vi "Stereo - IMAQ PrivGetCalibrationImageSampleInfo.vi"(8 "error in (no error)":errorcluster, 9 "Options":T3, 10 "Index":i32, 11 "Template Image":T4) -> (0 "error out":errorcluster, 1 "Undistorted Points":cluster{"X":dbl, "Y":dbl}[](array[cluster]), 2 "Back Projected Points":cluster{"X":dbl, "Y":dbl}[](array[cluster]), 3 "Reference Points":T1, 5 "Euler Angles":cluster{"X":dbl, "Y":dbl, "Z":dbl})   [LabVIEW 2014]
doc: "Returns information on the template image."
uses:
  <vilib>/vision/Image Controls.llb/IMAQ Image.ctl
  <vilib>/vision/Calibration.llb/Calibration Reference Points.ctl
  nivision.dll
panel:
  # "Overview: Returns information on the template image."
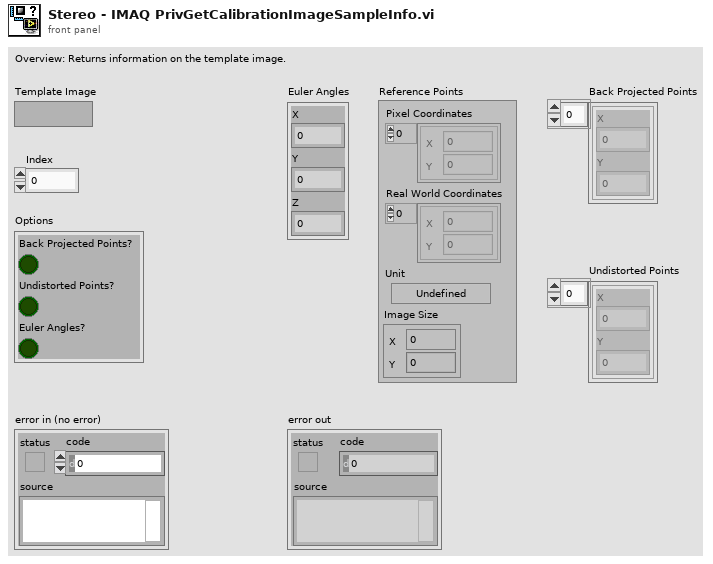
[diagram p1: front panel]
types:
  T1 = typedef "Calibration Reference Points.ctl" = cluster{"Pixel Coordinates":cluster{"X":dbl, "Y":dbl}[], "Real World Coordinates":cluster{"X":dbl, "Y":dbl}[], "Unit":T2, "Image Size":cluster{"X":u32, "Y":u32}}
  T2 = typedef "Image Unit" = enum32{"Undefined", "Angström", "Micrometer", "Millimeter", "Centimeter", "Meter", "Kilometer", "Microinch", "Inch", "Feet", "Nautical miles", "Standard miles", "Steps"}
  T3 = cluster{"Back Projected Points?":bool, "Undistorted Points?":bool, "Euler Angles?":bool}
  T4 = typedef "IMAQ Image.ctl" = refnum<image>
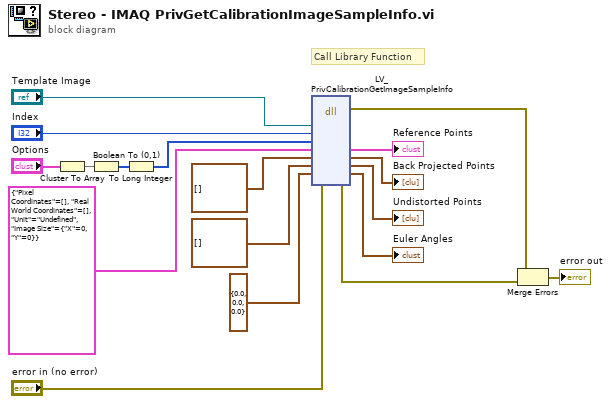
[diagram p0: block diagram]
diagram:
  # "Call Library Function"
  n1 = Cluster To Array(cluster="Options") -> (array=w9:bool[])
  n2 = Boolean To (0,1)(Boolean=w9) -> (0, 1=w7:i16[])
  n3 = To Long Integer(number=w7) -> (32bit integer=w6:i32[])
  n4 = dll-call lib="nivision.*" fn="LV_PrivCalibrationGetImageSampleInfo"("srcImage"="Template Image", "index"="Index", "options"=w6, "pixel points"=T1 {"Pixel Coordinates"=[], "Real World Coordinates"=[], "Unit"=enum."Undefined", "Image Size"={"X"=0, "Y"=0}} ("Reference Points"), "back projected points"=cluster{"X":dbl, "Y":dbl}[] [] ("Back Projected Points"), "undistorted points"=cluster{"X":dbl, "Y":dbl}[] [] ("Back Projected Points"), "euler angles"=cluster{"X":dbl, "Y":dbl, "Z":dbl} {"X"=0.0, "Y"=0.0, "Z"=0.0} ("Euler Angles"), "errorCluster"="error in (no error)") -> (error out=w3:errorcluster, "pixel points"=→"Reference Points":T1, "back projected points"=→"Back Projected Points":cluster{"X":dbl, "Y":dbl}[], "undistorted points"=→"Undistorted Points":cluster{"X":dbl, "Y":dbl}[], "euler angles"=→"Euler Angles":cluster{"X":dbl, "Y":dbl, "Z":dbl}, "errorCluster"=w2:errorcluster)  [unwired: 6 in, 2 out]
  n5 = Merge Errors(w3, w2) -> (→"error out":errorcluster)
